vi "Test FSM Editor.vi"() -> ()   [LabVIEW 2020]
uses:
  FSM Editor/FSM Editor.xctl
  Classes/FSM.Graph/FSM.Graph.lvclass
  Classes/FSM.Annotation/Annotation Style.ctl
  Classes/FSM.Annotation/FSM.Annotation.lvclass
panel:
  in  "Annotate":bool
  in  "Action Button":bool
  in  "Write Button":bool
  in  "Read Button":bool
  in  "stop":bool
  in  "FSM Editor":refnum<class "FSM.Graph.lvclass">(xcontrol)
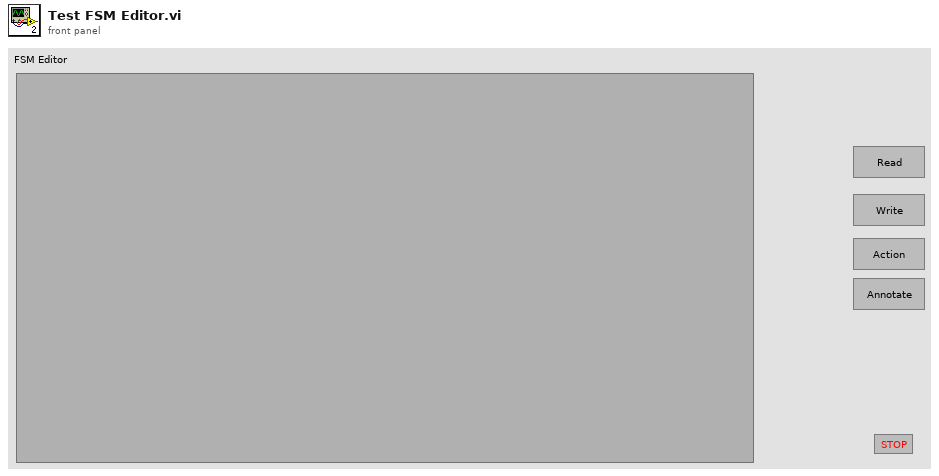
[diagram p1: front panel]
types:
  T1 = typedef "FSM.Annotation.lvclass/Annotation Style.ctl" = enum16{"Plain", "On", "Off", "On-Off"}
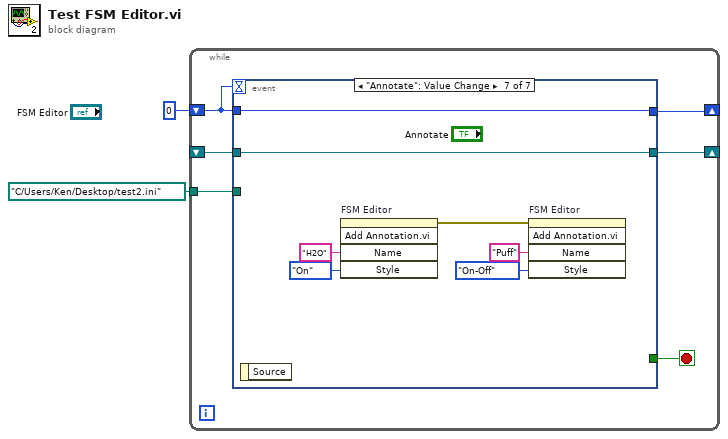
[diagram p0: block diagram]
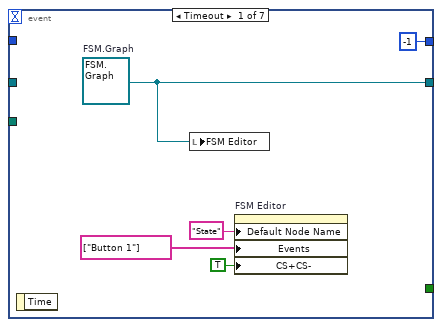
[diagram p2: hidden frame]
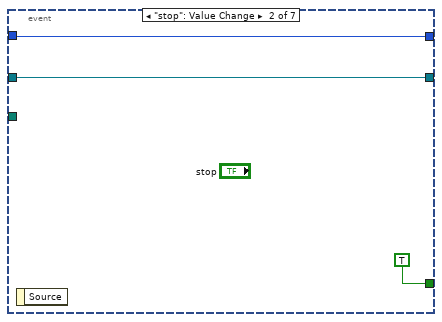
[diagram p3: hidden frame]
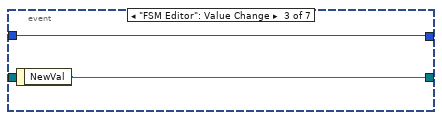
[diagram p4: hidden frame]
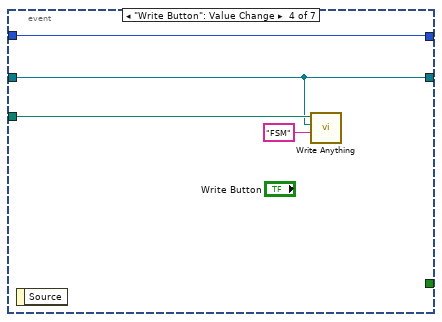
[diagram p5: hidden frame]
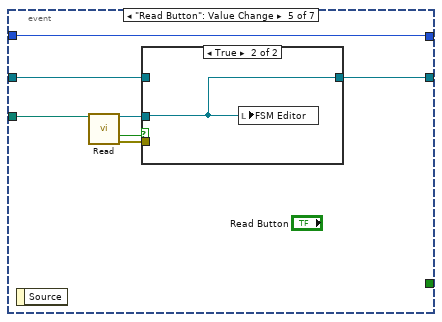
[diagram p6: hidden frame]
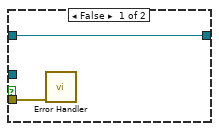
[diagram p7: hidden frame]
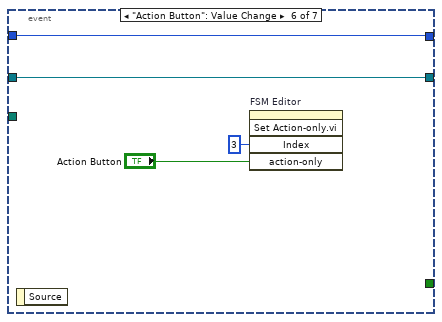
[diagram p8: hidden frame]
diagram:
  n1 = while {
    shift-right: [w6] -> _
    shift-left: 0 -> [w7]
    shift-right: [w5] -> _
    shift-left: _ -> [w4]
    tunnel: path "C:/Users/Ken/Desktop/test2.ini" -> [w3]
    stop <- w8 stop-if-true
    n2 = event shown="[6] \"Annotate\": Value Change" {
      selector: _ -> [_ _ _ _ _ _ _]
      dyn-events: _ -> [_ _ _ _ _ _ _]
      timeout: w7 -> [_ _ _ _ _ _ _]
      tunnel: [_ TRUE _ _ _ _ _] -> w8
      tunnel: w7 -> [_ w15 w18 w22 w29 w36 w43]
      tunnel: [-1 w15 w18 w22 w29 w36 w43] -> w6
      tunnel: [w11 w14 w17 w20 w27 w35 w42] -> w5
      tunnel: w4 -> [_ w14 _ w20 w28 w35 w42]
      tunnel: w3 -> [_ _ _ w21 w26 _ _]
      event Timeout {
        w11 = refnum<class "FSM.Graph.lvclass"> refnum  # FSM.Graph
        n3 = event-data() -> ()  [unwired: 1 in, 1 out]
        n4 = local write "FSM Editor"(w11) -> ()
        n5 = property on="FSM Editor" class="FSMGraph (strict)"("Default Node Name"="State", "Events"=string[] ["Button 1"], "CS+CS-"=TRUE) -> ()  [unwired: 2 in, 2 out]
      }
      event "stop": Value Change {
        n6 = event-data() -> ()  [unwired: 1 in, 1 out]
      }
      event "FSM Editor": Value Change {
        n7 = event-data() -> ("NewVal"=w17:refnum<class "FSM.Graph.lvclass">)  [unwired: 1 in]
      }
      event "Write Button": Value Change {
        n8 = event-data() -> ()  [unwired: 1 in, 1 out]
        n9 = call "Write Anything.vi"("Section Name (Name of \"Anything\")"="FSM" ("Section Name (Name of \"Anything\")"), "Anything"=w20, "Path (dialog)"=w21) -> ()  [unwired: 7 in, 2 out]
      }
      event "Read Button": Value Change {
        n10 = event-data() -> ()  [unwired: 1 in, 1 out]
        n11 = call "Read.vi"("Path"=w26) -> ("FSM.Graph"=w23:refnum<class "FSM.Graph.lvclass">, "Success"=w25:bool, "error out"=w24:errorcluster)  [unwired: 12 in]
        n12 = case shown="True" w25 {
          tunnel: w28 -> [w31 _]
          tunnel: [w31 w32] -> w27
          tunnel: w24 -> [w30 _]
          tunnel: w23 -> [_ w32]
          frame False {
            n13 = call "Error Handler.vi"("error in (no error)"=w30) -> ()  [unwired: 13 in, 2 out]
          }
          frame True {
            n14 = local write "FSM Editor"(w32) -> ()
          }
        }
      }
      event "Action Button": Value Change {
        n15 = event-data() -> ()  [unwired: 1 in, 1 out]
        n16 = invoke on="FSM Editor" class="FSM Editor (strict)" method="Set Action-only.vi"("Index"=3, "action-only"="Action Button") -> ()  [unwired: 3 in, 5 out]
      }
      event "Annotate": Value Change {
        n17 = event-data() -> ()  [unwired: 1 in, 1 out]
        n18 = invoke on="FSM Editor" class="FSM Editor (strict)" method="Add Annotation.vi"("Name"="H2O", "Style"=Annotation_Style."On") -> (error out=w39:errorcluster)  [unwired: 3 in, 4 out]
        n19 = invoke on="FSM Editor" class="FSM Editor (strict)" method="Add Annotation.vi"(error in=w39, "Name"="Puff", "Style"=Annotation_Style."On-Off") -> ()  [unwired: 2 in, 5 out]
      }
    }
  }
